vi "set_clock_enabled_state.vi"(8 "error in (no error)":errorcluster, 10 "enable clocks?":bool, 11 "FPGAWrapperMH120124FrameScan_PXI7813R in":refnum<class "FPGAWrapperMH120124FrameScan_PXI7813R.lvclass">) -> (0 "error out":errorcluster, 3 "FPGAWrapperMH120124FrameScan_PXI7813R out":refnum<class "FPGAWrapperMH120124FrameScan_PXI7813R.lvclass">)   [LabVIEW 2010, in "FPGAWrapperMH120124FrameScan_PXI7813R.lvclass"]
uses:
  FPGAWrapperMH120124FrameScan_PXI7813R.lvclass
  GenericFPGAWrapper/GenericFPGAWrapper/GenericFPGAWrapper.lvclass
  FPGAWrapperMH120124FrameScan_PXI7813R.lvclass/FPGAWrapperMH120124FrameScan_PXI7813R.ctl
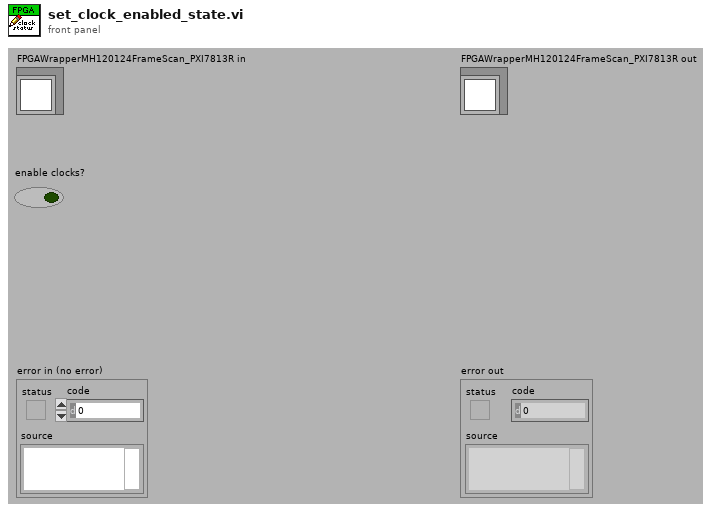
[diagram p1: front panel]
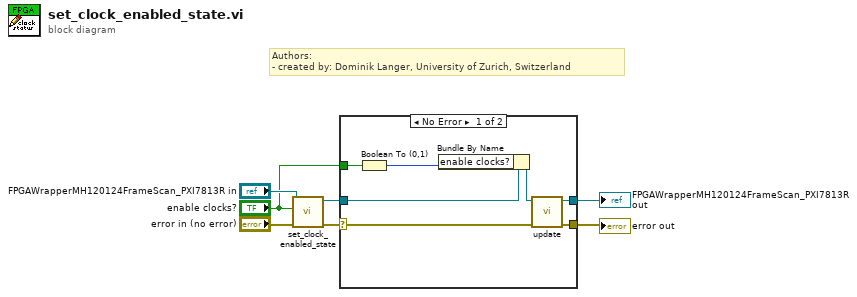
[diagram p0: block diagram]
diagram:
  # "Authors: \n- created by: Dominik Langer, University of Zurich, Switzerland"
  n1 = call-parent "set_clock_enabled_state.vi"("error in (no error)"="error in (no error)", "enable clocks?"="enable clocks?", "GenericFPGAWrapper in"="FPGAWrapperMH120124FrameScan_PXI7813R in") -> ("error out"=w5:errorcluster, "GenericFPGAWrapper out"=w4:refnum<class "FPGAWrapperMH120124FrameScan_PXI7813R.lvclass">)  [unwired: 7 in]
  n2 = case shown="No Error" w5 {
    selector: w5 -> [w11 w15]
    tunnel: w4 -> [w14 w16]
    tunnel: "enable clocks?" -> [w13 _]
    tunnel: [w9 w16] -> w2
    tunnel: [w10 w15] -> w1
    frame No Error {
      n3 = Boolean To (0,1)(Boolean=w13) -> (0, 1=w8:i16)
      n4 = Bundle By Name(cluster=w14, "enable clocks?"=w8) -> (w12:refnum<class "FPGAWrapperMH120124FrameScan_PXI7813R.lvclass">)
      n5 = call-dynamic "update.vi"("error in (no error)"=w11, "FPGAWrapperMH120124FrameScan_PXI7813R in"=w12) -> ("error out"=w10:errorcluster, "FPGAWrapperMH120124FrameScan_PXI7813R out"=w9:refnum<class "FPGAWrapperMH120124FrameScan_PXI7813R.lvclass">)  [unwired: 8 in]
    }
    frame Error {
    }
  }
  "error out" <- w1
  "FPGAWrapperMH120124FrameScan_PXI7813R out" <- w2
